vi "IntegrierenGV.vi"(0 "Probenvol.1":dbl, 1 "Integrieren1":bool, 2 "Integral1":dbl, 3 "Probenvol.2":dbl, 4 "Integrieren2":bool, 5 "Integral2":dbl, 6 "Int.Start1":dbl, 8 "Int.Stop1":dbl, 10 "Int.Start2":dbl, 11 "HorstProbenflußNr.":i32, 12 "Int.Stop2":dbl) -> (14 "Probenvol.1":dbl, 15 "Integrieren1":bool, 16 "Integral1":dbl, 17 "Probenvol.2":dbl, 18 "Integrieren2":bool, 19 "Integral2":dbl)   [LabVIEW 2010]
uses:
  GVMWHorst.vi
panel:
  in  "Big Ben, Methodenzeit, Zykluszeit0, Zykluszeit1, Zykluszeit2A, Zykluszeit2B":dbl[](array[numeric])
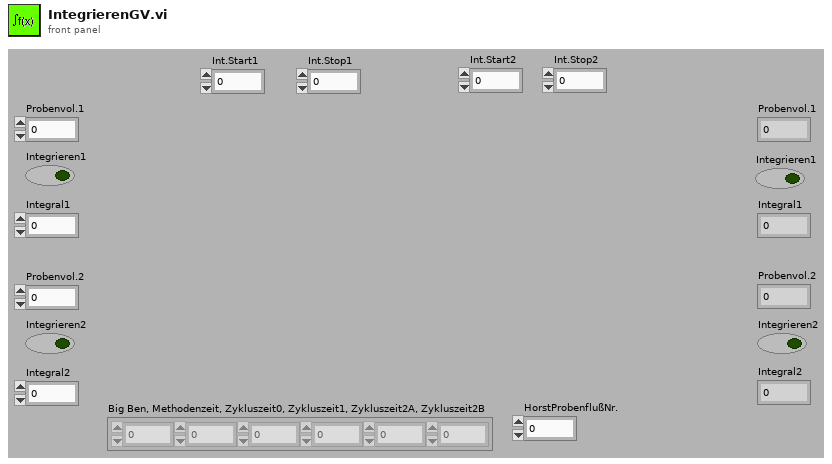
[diagram p1: front panel]
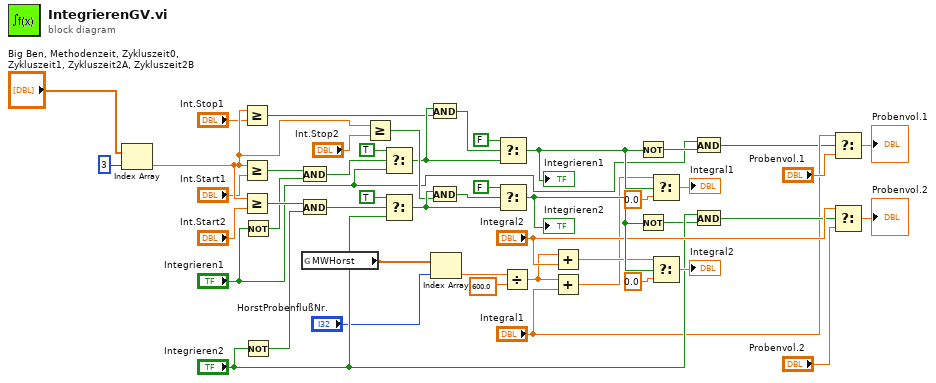
[diagram p0: block diagram]
diagram:
  n1 = Index Array(array="Big Ben, Methodenzeit, Zykluszeit0, Zykluszeit1, Zykluszeit2A, Zykluszeit2B", index=3 ("Index")) -> (element=w41:dbl)
  n2 = Greater Or Equal?(x=w41, y="Int.Stop1") -> (x >= y?=w12:bool)
  n3 = Greater Or Equal?(x=w41, y="Int.Start1") -> (x >= y?=w9:bool)
  n4 = Greater Or Equal?(x=w41, y="Int.Start2") -> (x >= y?=w29:bool)
  n5 = Not(x="Integrieren1") -> (.not. x?=w8:bool)
  n6 = Not(x="Integrieren2") -> (.not. x?=w28:bool)
  n7 = And(x=w9, y=w8) -> (x .and. y?=w10:bool)
  n8 = And(x=w29, y=w28) -> (x .and. y?=w30:bool)
  n9 = global read "GVMWHorst.vi" "MWHorst"() -> (w2:dbl[])
  n10 = Greater Or Equal?(x=w41, y="Int.Stop2") -> (x >= y?=w32:bool)
  n11 = Select(t=TRUE, s=w10, f="Integrieren1") -> (s? t:f=w16:bool)
  n12 = Select(t=TRUE, s=w30, f="Integrieren2") -> (s? t:f=w36:bool)
  n13 = And(x=w16, y=w12) -> (x .and. y?=w13:bool)
  n14 = And(x=w36, y=w32) -> (x .and. y?=w33:bool)
  n15 = Index Array(array=w2, index="HorstProbenflußNr.") -> (element=w4:dbl)
  n16 = Select(t=FALSE, s=w13, f=w16) -> (s? t:f=w21:bool)
  "Integrieren1" <- w21
  n17 = Select(t=FALSE, s=w33, f=w36) -> (s? t:f=w46:bool)
  "Integrieren2" <- w46
  n18 = Divide(x=w4, y=600.0) -> (x/y=w42:dbl)
  n19 = Add(x=w42, y="Integral2") -> (x+y=w37:dbl)
  n20 = Add(x=w42, y="Integral1") -> (x+y=w17:dbl)
  n21 = Not(x=w21) -> (.not. x?=w22:bool)
  n22 = Not(x=w46) -> (.not. x?=w39:bool)
  n23 = Select(t=w17, s=w21, f=0.0) -> (s? t:f=→"Integral1":dbl)
  n24 = Select(t=w37, s=w46, f=0.0) -> (s? t:f=→"Integral2":dbl)
  n25 = And(x="Integrieren1", y=w22) -> (x .and. y?=w23:bool)
  n26 = And(x="Integrieren2", y=w39) -> (x .and. y?=w40:bool)
  n27 = Select(t="Integral1", s=w23, f="Probenvol.1") -> (s? t:f=→"Probenvol.1":dbl)
  n28 = Select(t="Integral2", s=w40, f="Probenvol.2") -> (s? t:f=→"Probenvol.2":dbl)
